vi "Progetto_AnalisiDimensionale.vi"() -> ()   [LabVIEW 2020]
panel:
  in  "Saving File Path":path
  out "Stuck_Alarm":bool caption="Time has Elapsed"
  out "SPEED [m/s]":dbl
  out "LENGTH [mm]":dbl
  in  "Trigger_S2":bool
  in  "Trigger_S1":bool
  in  "STOP":bool
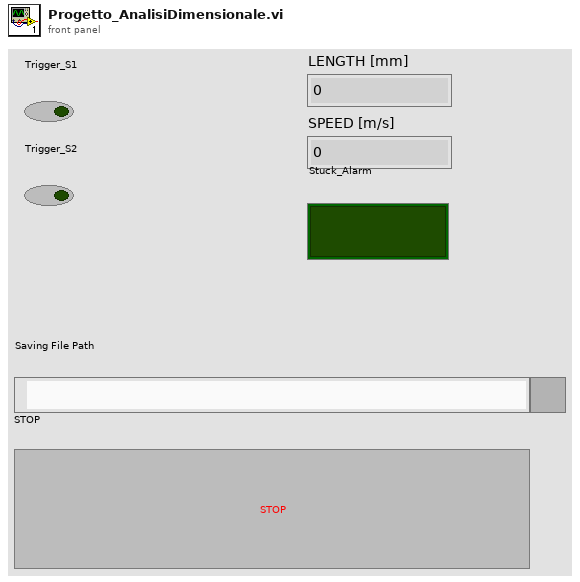
[diagram p1: front panel]
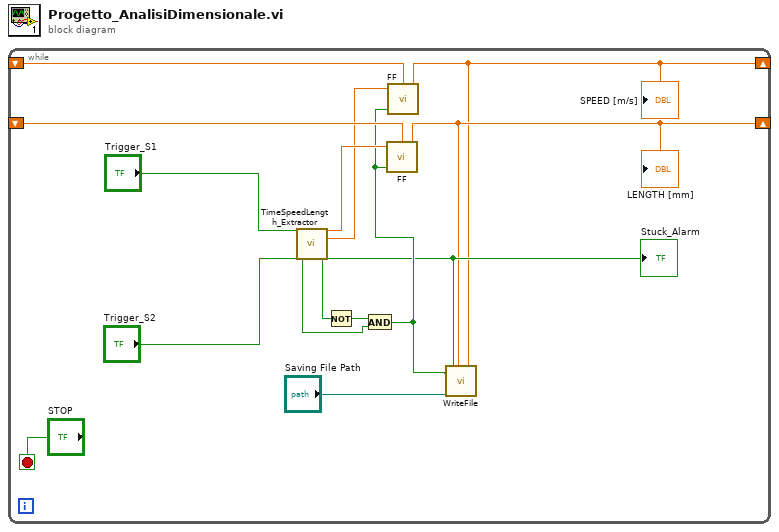
[diagram p0: block diagram]
diagram:
  n1 = while {
    shift-right: [w4] -> _
    shift-left: _ -> [w10]
    shift-right: [w3] -> _
    shift-left: _ -> [w7]
    stop <- "STOP" stop-if-true
    n2 = call "TimeSpeedLength_Extractor.vi"("TriggerS1"="Trigger_S1", "TriggerS2"="Trigger_S2") -> ("TriggerS2_prev-1"=w13:bool, "TriggerS2_prev0"=w1:bool, "Length   [mm]"=w9:dbl, "Speed [m/s]"=w8:dbl, "Stuck_Alarm"=w5:bool)  [unwired: 12 in, 9 out]
    "Stuck_Alarm" <- w5
    n3 = Not(x=w1) -> (.not. x?=w14:bool)
    n4 = And(x=w14, y=w13) -> (x .and. y?=w6:bool)
    n5 = call "FF.vi"("Q_prev"=w10, "Enable"=w6, "D"=w9) -> ("Q"=w4:dbl)  [unwired: 2 in]
    "LENGTH [mm]" <- w4
    n6 = call "FF.vi"("Q_prev"=w7, "Enable"=w6, "D"=w8) -> ("Q"=w3:dbl)  [unwired: 2 in]
    "SPEED [m/s]" <- w3
    n7 = call "WriteFile.vi"("Enable"=w6, "Saving File Path"="Saving File Path", "Alarm"=w5, "Length [mm]"=w4, "Speed [m/s]"=w3) -> ()  [unwired: 15 in]
  }
